vi "Full Force Test SAA.vi"(8 "error in (no error)":errorcluster, 10 "Model in":refnum<class "Model.lvclass">, 11 "Test Actuator State in":refnum<class "Test Actuator State.lvclass">) -> (0 "error out":errorcluster, 1 "Pass":bool, 2 "Model out":refnum<class "Model.lvclass">, 3 "Test Actuator State out":refnum<class "Test Actuator State.lvclass">)   [LabVIEW 2016]
uses:
  Model/Model/Model.lvclass
  Typedefs/ActuatorSetPoints.ctl
  <vilib>/platform/TimedLoop/XDataNode/XDataNode.xnode
  <vilib>/Platform/TimedLoop/XDataNode/nitl_modes.ctl
  <vilib>/Platform/TimedLoop/XDataNode/XDNodeRunTimeDep.lvlib
  <vilib>/Platform/TimedLoop/XDataNode/wakeup.ctl
  <vilib>/Platform/TimedLoop/XDataNode/timing_clust.ctl
  Test Actuator State.lvclass
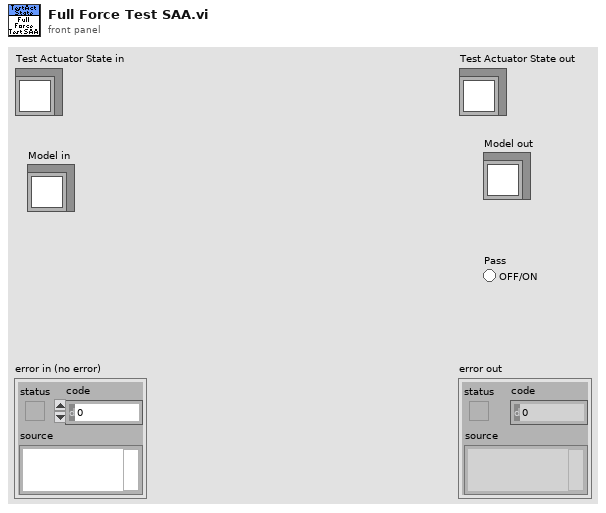
[diagram p1: front panel]
types:
  T1 = typedef "FullForceScanSettings.ctl" = cluster{"Force Tolerance (N)":dbl, "DAA Force Set Points":T2[], "Process Time (s)":dbl, "Sample Time (s)":dbl, "Max Moment (NM)":dbl, "SAA Force Set Points":T2[]}
  T2 = typedef "ForcePair.ctl" = cluster{"Axial Force":dbl, "Lateral Force":dbl}
  T3 = typedef "ActuatorSetPoints.ctl" = cluster{"Axial Force":dbl, "Lateral Force":dbl, "FC1 Force":dbl, "FC2 Force":dbl}
  T4 = typedef "XDNodeRunTimeDep.lvlib/timing_clust.ctl" = cluster{"Expected End [f-1]":u64, "Actual End [f-1]":u64, "Finished Late? [f-1]":bool, "Expected End [i-1]":u64, "Actual End [i-1]":u64, "Finished Late? [i-1]":bool, "Expected Start [i]":u64, "Actual Start [i]":u64, "Expected Start [f]":u64, "Actual Start [f]":u64, "Source Name":string, "Structure Name":string, "Period":i64, "Deadline":i64, "Offset":i64, "Start":i64, "Priority":i32, "Timeout":i32, "Mode":T5, "Wakeup Reason":T6, "Error":errorcluster, "Source Type":string, "Secondary Source Type":string, "Global End Time":u64, "Global Start Time":u64, "Frame Duration":u64, "Iteration Duration":u64, "Assigned CPU":i32, "I/O Scan Engine Mode":u32}
  T5 = typedef "XDNodeRunTimeDep.lvlib/nitl_modes.ctl" = enum32{"No Change", "Process missed periods, maintain original phase", "Discard missed periods, maintain original phase", "Process missed periods, ignore original phase", "Discard missed periods, ignore original phase"}
  T6 = typedef "XDNodeRunTimeDep.lvlib/wakeup.ctl" = enum32{"Normal", "Aborted", "Asynchronous wakeup", "Timing source error", "Timed loop error", "Timeout"}
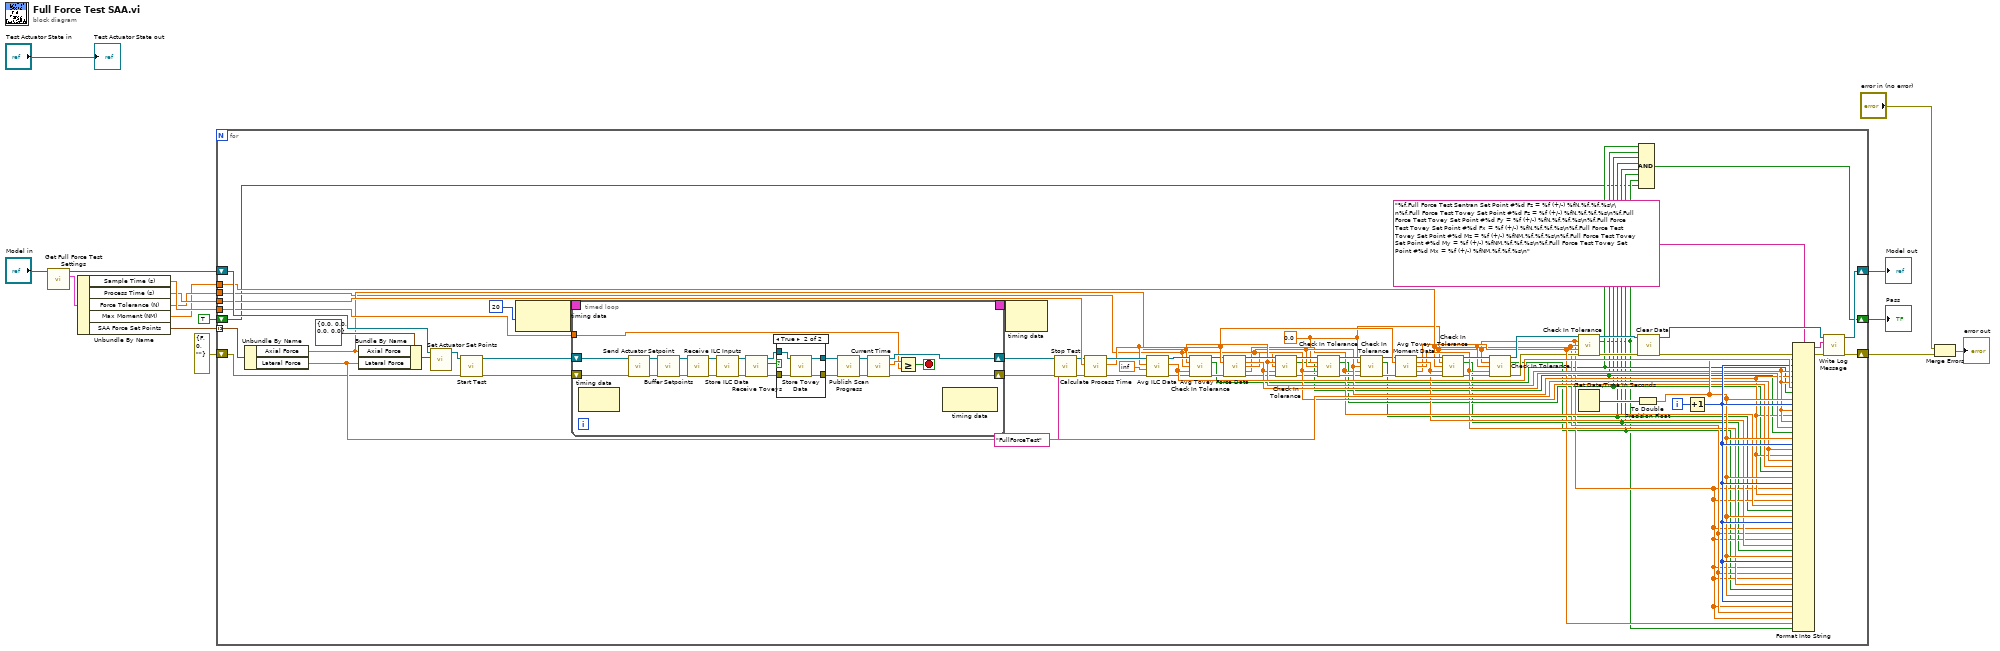
[diagram p0: block diagram]
diagram:
  n1 = call "Get Full Force Test Settings.vi"("Model in"="Model in") -> ("Full Force Test Settings"=w5:T1, "Model out"=w15:refnum<class "Model.lvclass">)  [unwired: 9 in]
  n2 = Unbundle By Name(w5) -> ("Sample Time (s)"=w14:dbl, "Process Time (s)"=w13:dbl, "Force Tolerance (N)"=w12:dbl, "Max Moment (NM)"=w7:dbl, "SAA Force Set Points"=w4:T2[])
  n3 = for {
    tunnel: w4 -> [w81] mode=indexing
    shift-right: [w86] -> w9
    shift-left: w15 -> [w89]
    tunnel: w14 -> [w88]
    tunnel: w13 -> [w76]
    tunnel: w12 -> [w60]
    shift-right: [w77] -> w8
    shift-left: errorcluster {"status"=FALSE, "code"=0, "source"=""} ("error out") -> [w22]
    tunnel: w7 -> [w42]
    shift-right: [w26] -> w1
    shift-left: TRUE -> [w27]
    i -> [w83]
    w41 = 0.0
    n4 = Unbundle By Name(w81) -> ("Axial Force"=w66:dbl, "Lateral Force"=w63:dbl)
    n5 = Bundle By Name(cluster=T3 {"Axial Force"=0.0, "Lateral Force"=0.0, "FC1 Force"=0.0, "FC2 Force"=0.0} ("Actuator Set Points"), "Axial Force"=w66, "Lateral Force"=w63) -> (w82:T3)
    n6 = call "Set Actuator Set Points.vi"("Actuator Set Points"=w82, "Model in"=w89) -> ("Model out"=w25:refnum<class "Model.lvclass">)  [unwired: 9 in]
    n7 = call "Start Test.vi"("error in (no error)"=w22, "Model in"=w25) -> ("error out"=w23:errorcluster, "Model out"=w24:refnum<class "Model.lvclass">)  [unwired: 8 in]
    n8 = node-c288(i64 20 ("Period")) -> (w37:T4)
    n9 = timed-loop {
      shift-right: [w110] -> w21
      shift-left: w24 -> [w112]
      shift-right: [w109] -> w20
      shift-left: w23 -> [w111]
      tunnel: w88 -> [w107]
      timing: w37 -> [_]
      timing-out: [_] -> w36
      stop <- w106 stop-if-true
      n10 = node-c288() -> ()  [unwired: 1 in, 1 out]
      n11 = call "Send Actuator Setpoint.vi"("error in (no error)"=w111, "Model in"=w112) -> ("error out"=w92:errorcluster, "Model out"=w94:refnum<class "Model.lvclass">)  [unwired: 8 in]
      n12 = call "Buffer Setpoints.vi"("error in (no error)"=w92, "Model in"=w94) -> ("error out"=w91:errorcluster, "Model out"=w93:refnum<class "Model.lvclass">)  [unwired: 8 in]
      n13 = call "Receive ILC Inputs.vi"("error in (no error)"=w91, "Model in"=w93) -> ("error out"=w95:errorcluster, "Model out"=w96:refnum<class "Model.lvclass">)  [unwired: 8 in]
      n14 = call "Store ILC Data.vi"("error in (no error)"=w95, "Model in"=w96) -> ("error out"=w104:errorcluster, "Model out"=w105:refnum<class "Model.lvclass">)  [unwired: 8 in]
      n15 = call "Receive Toveys.vi"("error in (no error)"=w104, "Model in"=w105) -> ("error out"=w102:errorcluster, "Data Received"=w101:bool, "Model out"=w103:refnum<class "Model.lvclass">)  [unwired: 7 in]
      n16 = case shown="True" w101 {
        tunnel: w103 -> [w116 w120]
        tunnel: w102 -> [w115 w119]
        tunnel: [w115 w118] -> w97
        tunnel: [w116 w117] -> w100
        frame False {
        }
        frame True {
          n17 = call "Store Tovey Data.vi"("error in (no error)"=w119, "Model in"=w120) -> ("error out"=w118:errorcluster, "Model out"=w117:refnum<class "Model.lvclass">)  [unwired: 8 in]
        }
      }
      n18 = call "Publish Scan Progress.vi"("error in (no error)"=w97, "Model in"=w100) -> ("error out"=w98:errorcluster, "Model out"=w99:refnum<class "Model.lvclass">)  [unwired: 8 in]
      n19 = call "Current Time.vi"("error in (no error)"=w98, "Model in"=w99) -> ("error out"=w109:errorcluster, "Time"=w108:dbl, "Model out"=w110:refnum<class "Model.lvclass">)  [unwired: 7 in]
      n20 = Greater Or Equal?(x=w108, y=w107) -> (x >= y?=w106:bool)
      n21 = node-c288() -> ()  [unwired: 1 in, 1 out]
    }
    n22 = node-c288(w36) -> ()  [unwired: 1 out]
    n23 = call "Stop Test.vi"("error in (no error)"=w20, "Test"="FullForceTest", "Model in"=w21) -> ("error out"=w19:errorcluster, "Model out"=w18:refnum<class "Model.lvclass">)  [unwired: 7 in]
    n24 = call "Calculate Process Time.vi"("error in (no error)"=w19, "Seconds"=w76, "Model in"=w18) -> ("error out"=w74:errorcluster, "Time"=w73:dbl, "Model out"=w75:refnum<class "Model.lvclass">)  [unwired: 6 in]
    n25 = call "Avg ILC Data.vi"("error in (no error)"=w74, "Before This Time"=inf, "After This Time"=w73, "Model in"=w75) -> ("error out"=w70:errorcluster, "Force"=w71:dbl, "Model out"=w72:refnum<class "Model.lvclass">)  [unwired: 5 in]
    n26 = call "Check In Tolerance.vi"("Model in"=w72, "Expected"=w66, "Tolerance"=w60, "Actual"=w71, "error in (no error)"=w70) -> ("Model out"=w40:refnum<class "Model.lvclass">, "Pass"=w34:bool, "error out"=w39:errorcluster)  [unwired: 8 in]
    n27 = call "Avg Tovey Force Data.vi"("Model in"=w40, "After This Time"=w73, "error in (no error)"=w39) -> ("Model out"=w67:refnum<class "Model.lvclass">, "Fz"=w65:dbl, "Fy"=w62:dbl, "Fx"=w52:dbl, "error out"=w59:errorcluster)  [unwired: 8 in]
    n28 = call "Check In Tolerance.vi"("Model in"=w67, "Expected"=w66, "Tolerance"=w60, "Actual"=w65, "error in (no error)"=w59) -> ("Model out"=w64:refnum<class "Model.lvclass">, "Pass"=w33:bool, "error out"=w58:errorcluster)  [unwired: 8 in]
    n29 = call "Check In Tolerance.vi"("Model in"=w64, "Expected"=w41, "Tolerance"=w60, "Actual"=w62, "error in (no error)"=w58) -> ("Model out"=w61:refnum<class "Model.lvclass">, "Pass"=w32:bool, "error out"=w57:errorcluster)  [unwired: 8 in]
    n30 = call "Check In Tolerance.vi"("Model in"=w61, "Expected"=w41, "Tolerance"=w60, "Actual"=w52, "error in (no error)"=w57) -> ("Model out"=w55:refnum<class "Model.lvclass">, "Pass"=w31:bool, "error out"=w56:errorcluster)  [unwired: 8 in]
    n31 = call "Avg Tovey Moment Data.vi"("Model in"=w55, "After This Time"=w73, "error in (no error)"=w56) -> ("Model out"=w54:refnum<class "Model.lvclass">, "Mz"=w51:dbl, "My"=w48:dbl, "Mx"=w47:dbl, "error out"=w53:errorcluster)  [unwired: 8 in]
    n32 = call "Check In Tolerance.vi"("Model in"=w54, "Expected"=w41, "Tolerance"=w42, "Actual"=w51, "error in (no error)"=w53) -> ("Model out"=w50:refnum<class "Model.lvclass">, "Pass"=w30:bool, "error out"=w45:errorcluster)  [unwired: 8 in]
    n33 = call "Check In Tolerance.vi"("Model in"=w50, "Expected"=w41, "Tolerance"=w42, "Actual"=w48, "error in (no error)"=w45) -> ("Model out"=w49:refnum<class "Model.lvclass">, "Pass"=w29:bool, "error out"=w44:errorcluster)  [unwired: 8 in]
    n34 = call "Check In Tolerance.vi"("Model in"=w49, "Expected"=w41, "Tolerance"=w42, "Actual"=w47, "error in (no error)"=w44) -> ("Model out"=w46:refnum<class "Model.lvclass">, "Pass"=w28:bool, "error out"=w43:errorcluster)  [unwired: 8 in]
    n35 = Get Date/Time In Seconds() -> (seconds since 1Jan1904=w84:timestamp)
    n36 = To Double Precision Float(number=w84) -> (double precision float=w68:dbl)
    n37 = call "Clear Data.vi"("error in (no error)"=w43, "Model in"=w46) -> ("error out"=w79:errorcluster, "Model out"=w87:refnum<class "Model.lvclass">)  [unwired: 8 in]
    n38 = Compound Arithmetic op=AND(w34, w33, w32, w31, w30, w29, w28, w27) -> (w26:bool)
    n39 = Increment(x=w83) -> (x+1=w69:i32)
    n40 = Format Into String(format string="%f,Full Force Test Sentran Set Point #%d Fz = %f (+/-) %fN,%f,%f,%s\r\n%f,Full Force Test Tovey Set Point #%d Fz = %f (+/-) %fN,%f,%f,%s\n%f,Full Force Test Tovey Set Point #%d Fy = %f (+/-) %fN,%f,%f,%s\n%f,Full Force Test Tovey Set Point #%d Fx = %f (+/-) %fN,%f,%f,%s\n%f,Full Force Test Tovey Set Point #%d Mz = %f (+/-) %fNM,%f,%f,%s\n%f,Full Force Test Tovey Set Point #%d My = %f (+/-) %fNM,%f,%f,%s\n%f,Full Force Test Tovey Set Point #%d Mx = %f (+/-) %fNM,%f,%f,%s\n", error in=w79, w68, w69, w66, w60, w66, w71, w34, w68, w69, w66, w60, w66, w65, w33, w68, w69, w63, w60, w63, w62, w32, w68, w69, w41, w60, w41, w52, w31, w68, w69, w41, w42, w41, w51, w30, w68, w69, w41, w42, w41, w48, w29, w68, w69, w41, w42, w41, w47, w28) -> (resulting string=w80:string, error out=w78:errorcluster)  [unwired: 1 in]
    n41 = call "Write Log Message.vi"("error in (no error)"=w78, "Message"=w80, "Model in"=w87) -> ("error out"=w77:errorcluster, "Model out"=w86:refnum<class "Model.lvclass">)  [unwired: 7 in]
  }
  "Model out" <- w9
  "Pass" <- w1
  n42 = Merge Errors("error in (no error)", w8) -> (→"error out":errorcluster)
  "Test Actuator State out" <- "Test Actuator State in"
